vi "1. deney.vi"() -> ()   [LabVIEW 2020]
uses:
  <vilib>/measure/NI_MAPro.lvlib
  <vilib>/measure/maspectr.llb/FFT Spectrum (Mag-Phase) for 1 Chan.vi
panel:
  out "Waveform Graph 2":cluster{"f0":dbl, "df":dbl, "magnitude":dbl[]}(graph)
  out "Waveform Graph":dynamicdata(graph)
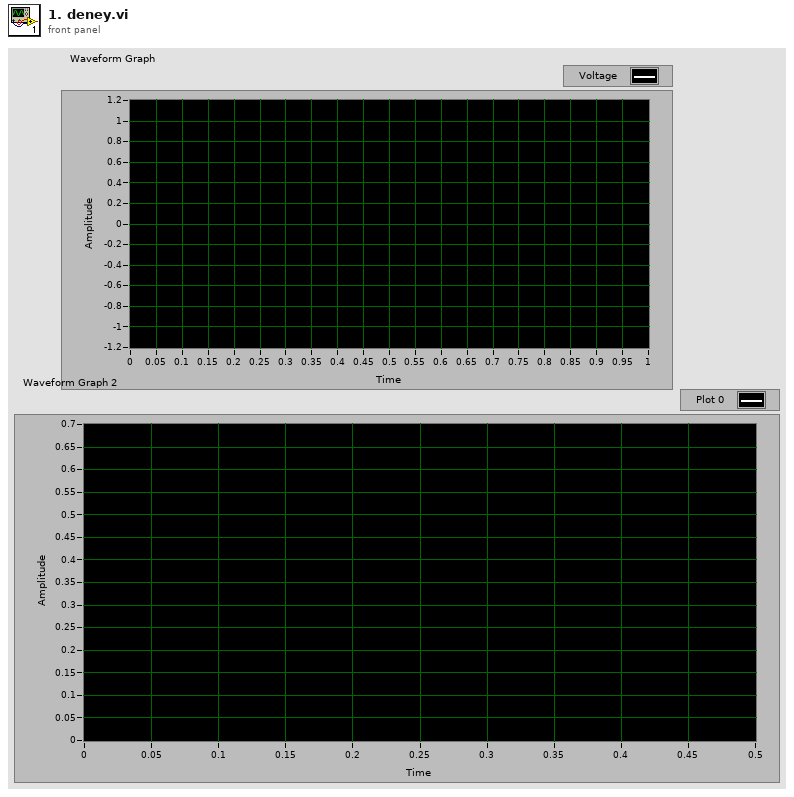
[diagram p1: front panel]
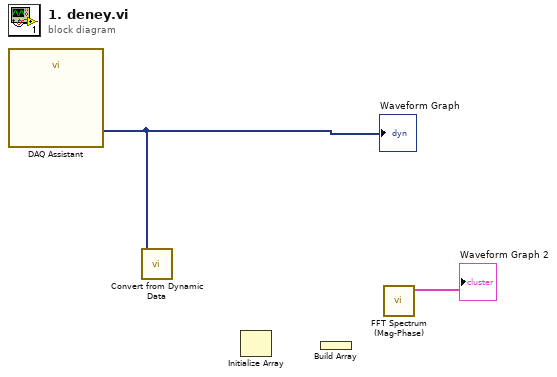
[diagram p0: block diagram]
diagram:
  n1 = call "DAQ Assistant"() -> ("data"=w2:dynamicdata)  [unwired: 17 in, 2 out]
  "Waveform Graph" <- w2
  n2 = call "Convert from Dynamic Data"("Dynamic Data Type"=w2) -> ()  [unwired: 3 in, 1 out]
  n3 = Initialize Array() -> ()  [unwired: 2 in, 1 out]
  n4 = Build Array() -> ()  [unwired: 1 in, 1 out]
  n5 = call-poly <vilib>:"FFT Spectrum (Mag-Phase).vi"() -> ("magnitude"=→"Waveform Graph 2":cluster{"f0":dbl, "df":dbl, "magnitude":dbl[]})  [unwired: 7 in, 4 out]
